vi "Math-Truncated Exponential PDF.vi"(0 "samples":i32, 5 "Min":dbl, 7 "Max":dbl, 9 "Lambda":dbl) -> (4 "X":dbl[](array[numeric]), 6 "PDF(X)":dbl[](array[numeric]))   [LabVIEW 2020]
uses:
  <vilib>/Analysis/1siggen.llb/Ramp Pattern by Samples.vi
  <vilib>/Analysis/NI_AALBase.lvlib
panel:
  out "XY Graph":cluster{"Ramp Pattern":dbl[], dbl[]}(graph)
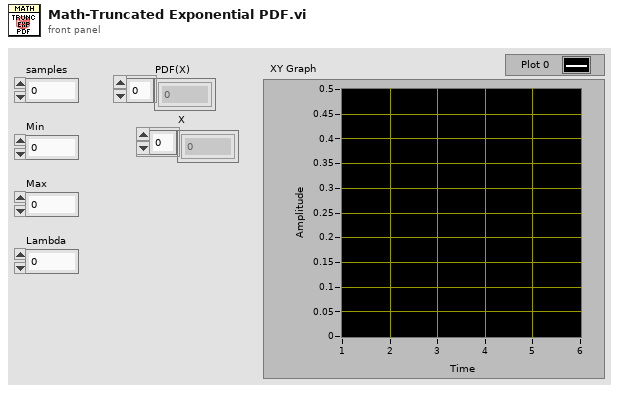
[diagram p1: front panel]
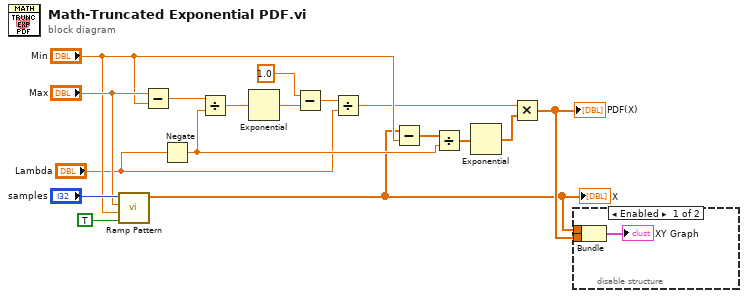
[diagram p0: block diagram]
diagram:
  n1 = call-poly <vilib>:"Ramp Pattern.vi"("exclude end?"=TRUE, "start"="Min", "end"="Max", "samples"="samples") -> ("Ramp Pattern"=w3:dbl[])  [unwired: 6 in, 1 out]
  "X" <- w3
  n2 = Subtract(x="Max", y="Min") -> (x-y=w17:dbl)
  n3 = Negate(x="Lambda") -> (-x=w7:dbl)
  n4 = Divide(x=w17, y=w7) -> (x/y=w16:dbl)
  n5 = Exponential(1:w16) -> (0:w15:dbl)
  n6 = Subtract(x=1.0, y=w15) -> (x-y=w14:dbl)
  n7 = Divide(x=w14, y="Lambda") -> (x/y=w1:dbl)
  n8 = Subtract(x=w3, y="Min") -> (x-y=w8:dbl[])
  n9 = Divide(x=w8, y=w7) -> (x/y=w6:dbl[])
  n10 = Exponential(1:w6) -> (0:w5:dbl[])
  n11 = Multiply(x=w1, y=w5) -> (x*y=w4:dbl[])
  "PDF(X)" <- w4
  n12 = disable-structure shown="Enabled" {
    disable-tunnel: w4 -> [w20 _]
    disable-tunnel: w3 -> [w19 _]
    frame Enabled {
      n13 = Bundle("Ramp Pattern"=w19, w20) -> (→"XY Graph":cluster{"Ramp Pattern":dbl[], dbl[]})  [unwired: 1 in]
    }
    frame Disabled {
    }
  }
